vi "14-sub.vi"(1 "n_Collatz":u64 min=1 step=1) -> (0 "(n+1)_Collatz":u64)   [LabVIEW 2021]
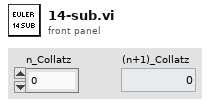
[diagram p1: front panel]
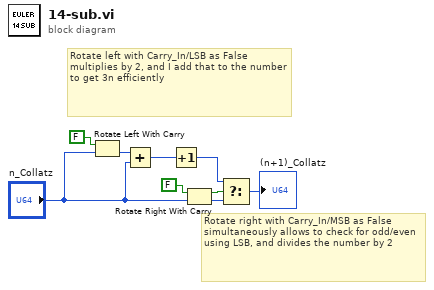
[diagram p0: block diagram]
diagram:
  # "Rotate left with Carry_In/LSB as False multiplies by 2, and I add that to the number to get 3n efficiently"
  # "Rotate right with Carry_In/MSB as False simultaneously allows to check for odd/even using LSB, and divides the number by 2"
  n1 = Rotate Left With Carry(2:"n_Collatz", 3:FALSE ("carry")) -> (0:w5:u64)  [unwired: 1 out]
  n2 = Add(x=w5, y="n_Collatz") -> (x+y=w4:u64)
  n3 = Increment(x=w4) -> (x+1=w1:u64)
  n4 = Rotate Right With Carry(2:"n_Collatz", 3:FALSE ("carry")) -> (0:w6:u64, 1:w9:bool)
  n5 = Select(t=w1, s=w9, f=w6) -> (s? t:f=→"(n+1)_Collatz":u64)
